vi "linear ramp.vi"(6 "# of Samples":sgl=10.0, 10 "Right Power In":i8=100, 11 "Left Power In":i8=100) -> (2 "Right Power Out":i8, 3 "Left Power out":i8)   [LabVIEW 2012, in "BlockParty4150.lvrbt"]
uses:
  BlockParty4150.lvrbt
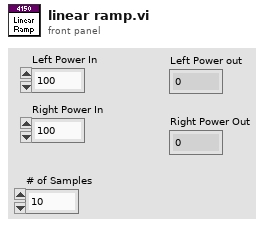
[diagram p1: front panel]
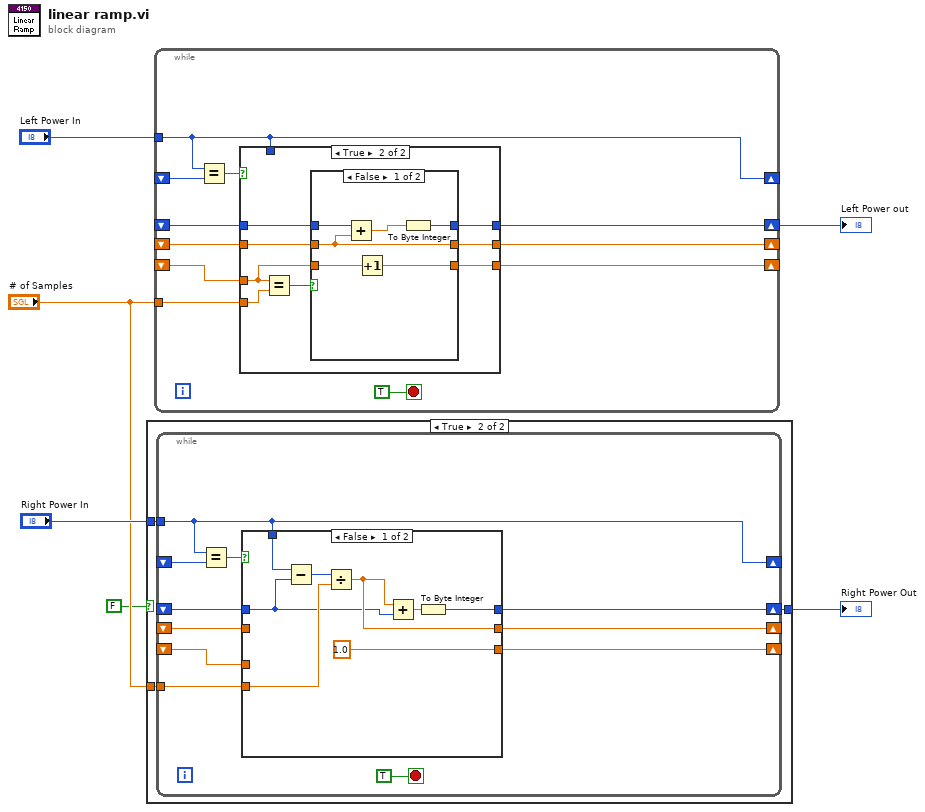
[diagram p0: block diagram]
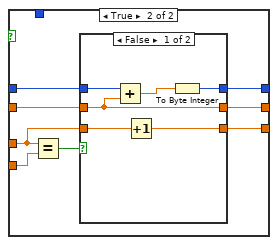
[diagram p3: hidden frame]
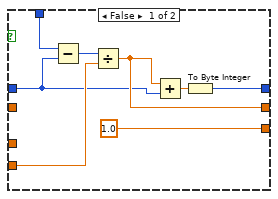
[diagram p5: hidden frame]
diagram:
  n1 = case shown="True" FALSE {
    tunnel: "Right Power In" -> [w7 w10]
    tunnel: "# of Samples" -> [_ w9]
    tunnel: [w7 w8] -> w2
    frame False {
    }
    frame True {
      n2 = while {
        tunnel: w9 -> [w17]
        tunnel: w10 -> [w12]
        shift-right: [w12] -> _
        shift-left: _ -> [w19]
        shift-right: [w13] -> _
        shift-left: _ -> [w14]
        shift-right: [w15] -> _
        shift-left: _ -> [w18]
        shift-right: [w16] -> w8
        shift-left: _ -> [w11]
        stop <- TRUE stop-if-true
        n3 = Equal?(x=w12, y=w19) -> (x = y?=w20:bool)
        n4 = case shown="False" w20 {
          tunnel: w18 -> [_ w34]
          tunnel: w17 -> [w27 w37]
          tunnel: [w25 w35] -> w16
          tunnel: [sgl 1.0 w33] -> w15
          tunnel: w14 -> [_ w32]
          tunnel: [w23 w31] -> w13
          tunnel: w12 -> [w29 _]
          tunnel: w11 -> [w22 w30]
          frame False {
            n5 = Subtract(x=w29, y=w22) -> (x-y=w28:i8)
            n6 = Divide(x=w28, y=w27) -> (x/y=w23:sgl)
            n7 = Add(x=w23, y=w22) -> (x+y=w24:sgl)
            n8 = To Byte Integer(number=w24) -> (8bit integer=w25:i8)
          }
          frame True {
            n9 = Equal?(x=w34, y=w37) -> (x = y?=w36:bool)
            n10 = case shown="False" w36 {
              tunnel: [w39 w44] -> w35
              tunnel: [w41 w46] -> w33
              tunnel: w34 -> [w42 w46]
              tunnel: [w40 w45] -> w31
              tunnel: w32 -> [w40 w45]
              tunnel: w30 -> [w38 w44]
              frame False {
                n11 = Add(x=w38, y=w40) -> (x+y=w43:sgl)
                n12 = Increment(x=w42) -> (x+1=w41:sgl)
                n13 = To Byte Integer(number=w43) -> (8bit integer=w39:i8)
              }
              frame True {
              }
            }
          }
        }
      }
    }
  }
  "Right Power Out" <- w2
  n14 = while {
    tunnel: "# of Samples" -> [w54]
    tunnel: "Left Power In" -> [w49]
    shift-right: [w49] -> _
    shift-left: _ -> [w56]
    shift-right: [w50] -> _
    shift-left: _ -> [w51]
    shift-right: [w52] -> _
    shift-left: _ -> [w55]
    shift-right: [w53] -> w5
    shift-left: _ -> [w48]
    stop <- TRUE stop-if-true
    n15 = Equal?(x=w49, y=w56) -> (x = y?=w47:bool)
    n16 = case shown="True" w47 {
      tunnel: w55 -> [_ w70]
      tunnel: w54 -> [w63 w73]
      tunnel: [w61 w71] -> w53
      tunnel: [sgl 1.0 w69] -> w52
      tunnel: w51 -> [_ w68]
      tunnel: [w59 w67] -> w50
      tunnel: w49 -> [w65 _]
      tunnel: w48 -> [w58 w66]
      frame False {
        n17 = Subtract(x=w65, y=w58) -> (x-y=w64:i8)
        n18 = Divide(x=w64, y=w63) -> (x/y=w59:sgl)
        n19 = Add(x=w59, y=w58) -> (x+y=w60:sgl)
        n20 = To Byte Integer(number=w60) -> (8bit integer=w61:i8)
      }
      frame True {
        n21 = Equal?(x=w70, y=w73) -> (x = y?=w72:bool)
        n22 = case shown="False" w72 {
          tunnel: [w75 w80] -> w71
          tunnel: [w77 w82] -> w69
          tunnel: w70 -> [w78 w82]
          tunnel: [w76 w81] -> w67
          tunnel: w68 -> [w76 w81]
          tunnel: w66 -> [w74 w80]
          frame False {
            n23 = Add(x=w74, y=w76) -> (x+y=w79:sgl)
            n24 = Increment(x=w78) -> (x+1=w77:sgl)
            n25 = To Byte Integer(number=w79) -> (8bit integer=w75:i8)
          }
          frame True {
          }
        }
      }
    }
  }
  "Left Power out" <- w5
